vi "WSVCAP SHL Host LL Manage Top Level Controls Core Gatekeeper.vi"(4 "FPGA":T2, 6 "Operation":T1, 8 "error in (no error)":errorcluster) -> (0 "error out":errorcluster)   [LabVIEW 2017]
uses:
  Type Defs/WSVCAP SHL FPGA Enum.ctl
  Type Defs/WSVCAP SHL Gatekeeper Operation Enum.ctl
  WSVCAP SHL Host LL I2C Semaphore Global.vi
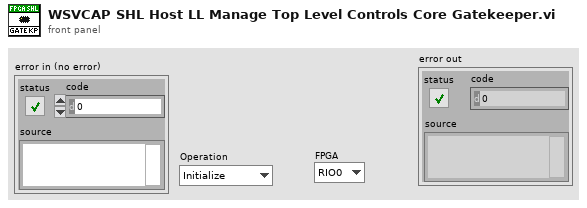
[diagram p1: front panel]
types:
  T1 = typedef "WSVCAP SHL Gatekeeper Operation Enum.ctl" = enum16{"Initialize", "Lock", "Unlock", "Close"}
  T2 = typedef "WSVCAP SHL FPGA Enum.ctl" = enum16{"RIO0", "RIO1"}
  T3 = typedef "Semaphore RefNum" = refnum<k1>
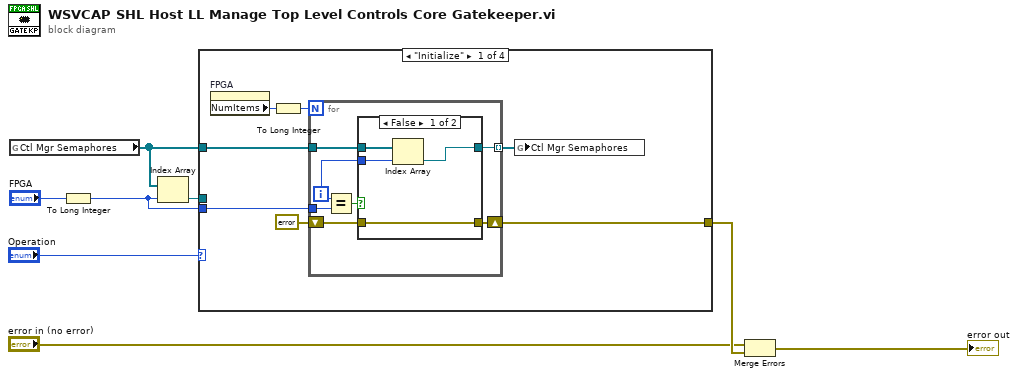
[diagram p0: block diagram]
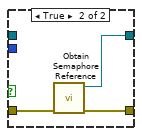
[diagram p2: hidden frame]
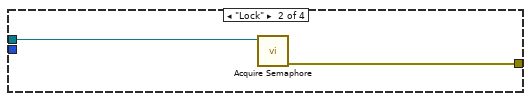
[diagram p3: hidden frame]
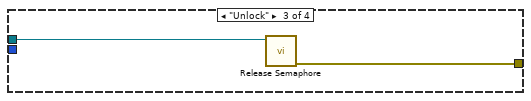
[diagram p4: hidden frame]
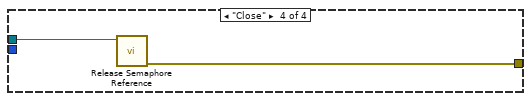
[diagram p5: hidden frame]
diagram:
  n1 = global read "WSVCAP SHL Host LL I2C Semaphore Global.vi" "Ctl Mgr Semaphores"() -> (w3:T3[])
  n2 = To Long Integer(number="FPGA") -> (32bit integer=w2:i32)
  n3 = Index Array(array=w3, index=w2) -> (element=w4:T3)
  n4 = case shown="\"Initialize\"" "Operation" {
    tunnel: w4 -> [_ w31 w33 w34]
    tunnel: [w12 w30 w32 w35] -> w6
    tunnel: w3 -> [w9 _ _ _]
    tunnel: w2 -> [w10 _ _ _]
    frame "Initialize" {
      n5 = property on="FPGA" class="Enum (strict)"() -> ("NumItems"=w14:u32)  [unwired: 2 in, 2 out]
      n6 = To Long Integer(number=w14) -> (32bit integer=w13:i32)
      n7 = for {
        N: w13 -> [_]
        shift-right: [w21] -> w12
        shift-left: errorcluster {"status"=FALSE, "code"=0, "source"=""} ("error out") -> [w20]
        tunnel: w10 -> [w19]
        tunnel: w9 -> [w17]
        tunnel: [w22] -> w11 mode=indexing
        i -> [w16]
        n8 = Equal?(x=w16, y=w19) -> (x = y?=w18:bool)
        n9 = case shown="False" w18 {
          tunnel: [w24 w27] -> w22
          tunnel: [w26 w29] -> w21
          tunnel: w20 -> [w26 w28]
          tunnel: w17 -> [w25 _]
          tunnel: w16 -> [w23 _]
          frame False {
            n10 = Index Array(array=w25, index=w23) -> (element=w24:T3)
          }
          frame True {
            n11 = call <vilib>:"Obtain Semaphore Reference.vi"("error in (no error)"=w28) -> ("error out"=w29:errorcluster, "semaphore"=w27:T3)  [unwired: 4 in, 1 out]
          }
        }
      }
      n12 = global write "WSVCAP SHL Host LL I2C Semaphore Global.vi" "Ctl Mgr Semaphores"(w11) -> ()
    }
    frame "Lock" {
      n13 = call <vilib>:"Acquire Semaphore.vi"("semaphore"=w31) -> ("error out"=w30:errorcluster)  [unwired: 4 in, 2 out]
    }
    frame "Unlock" {
      n14 = call <vilib>:"Release Semaphore.vi"("semaphore"=w33) -> ("error out"=w32:errorcluster)  [unwired: 5 in, 1 out]
    }
    frame "Close" {
      n15 = call <vilib>:"Release Semaphore Reference.vi"("semaphore"=w34) -> ("error out"=w35:errorcluster)  [unwired: 9 in, 1 out]
    }
  }
  n16 = Merge Errors("error in (no error)", w6) -> (→"error out":errorcluster)
